vi "Picture Rotation.vi"(6 "Mask Color (Black)":u32(colorbox), 8 "transparent?":bool, 9 "theta (deg)":dbl(slide) scale=-180.0..180.0, 10 "image data in":T2, 11 "Path":path) -> (2 "image data out":T2, 3 "Picture":picture)   [LabVIEW 2018]
uses:
  <vilib>/picture/picture.llb/imagedata.ctl
  <vilib>/Utility/miscctls.llb/LVBoundsTypeDef.ctl
panel:
  out "output cluster":T1
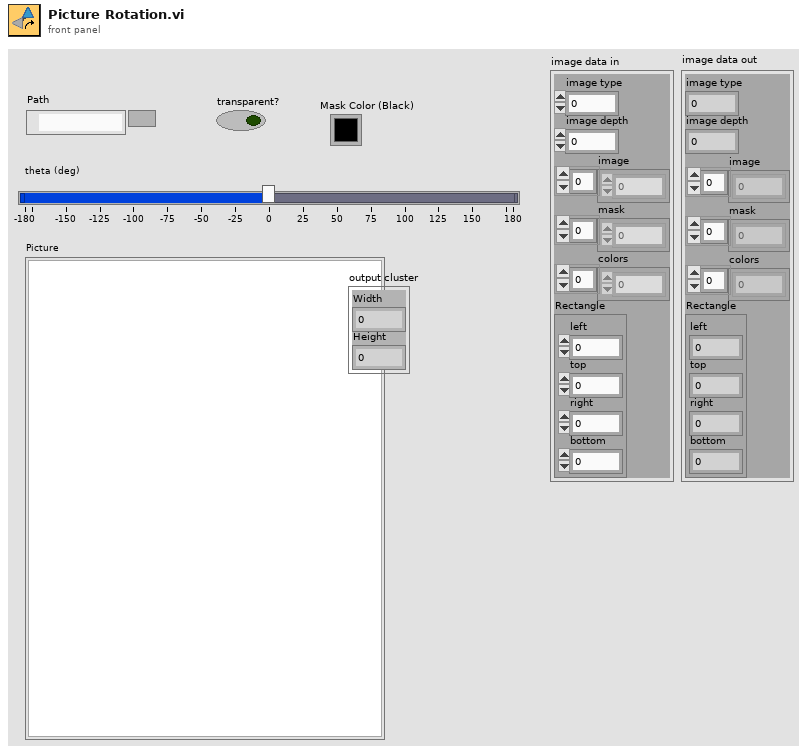
[diagram p1: front panel]
types:
  T1 = typedef "LVBoundsTypeDef.ctl" = cluster{"Width":u32, "Height":u32}
  T2 = typedef "imagedata.ctl" = cluster{"image type":i32, "image depth":i32, "image":u8[], "mask":u8[], "colors":u32[], "Rectangle":cluster{"left":i16, "top":i16, "right":i16, "bottom":i16}}
  T3 = cluster{"left":i16, "top":i16, "right":i16, "bottom":i16}
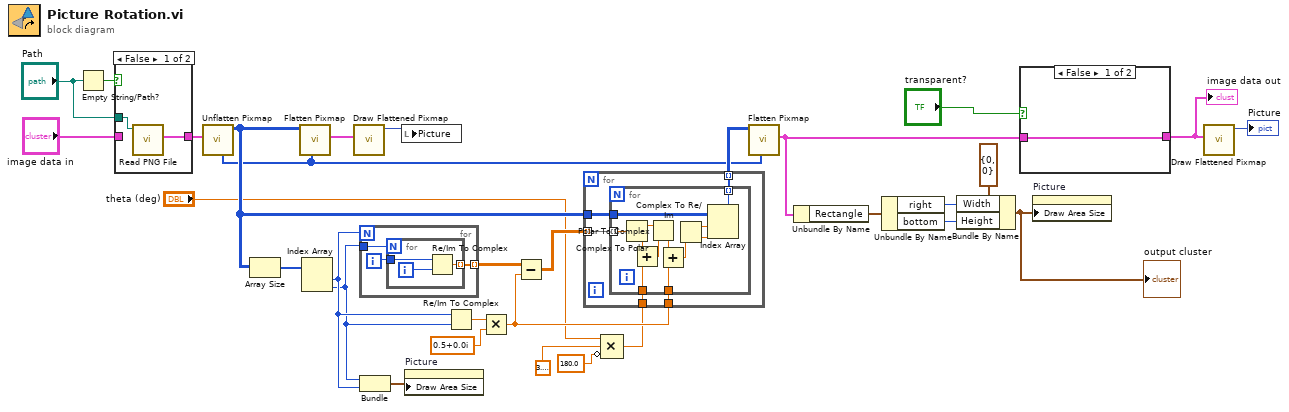
[diagram p0: block diagram]
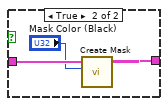
[diagram p2: hidden frame]
diagram:
  n1 = Empty String/Path?(string/path="Path") -> (empty?=w12:bool)
  n2 = case shown="False" w12 {
    tunnel: [w33 w34] -> w21
    tunnel: "Path" -> [w32 _]
    tunnel: "image data in" -> [_ w34]
    frame False {
      n3 = call <vilib>:"Read PNG File.vi"("path to PNG file"=w32) -> ("image data"=w33:T2)  [unwired: 8 in, 2 out]
    }
    frame True {
    }
  }
  n4 = call <vilib>:"Unflatten Pixmap.vi"("image data"=w21) -> ("24-bit pixmap"=w22:u32[][], "colors"=w19:u32[])  [unwired: 4 in, 5 out]
  n5 = Array Size(array=w22) -> (size(s)=w28:i32[])
  n6 = call <vilib>:"Flatten Pixmap.vi"("colors"=w19, "24-bit pixmap"=w22) -> ("image data"=w18:T2)  [unwired: 9 in]
  n7 = Index Array(array=w28) -> (element #1=w26:i32, element #2=w25:i32)  [unwired: 2 in]
  n8 = call <vilib>:"Draw Flattened Pixmap.vi"("image data"=w18) -> ("new picture"=w4:picture)  [unwired: 8 in]
  n9 = for {
    N: w26 -> [_]
    tunnel: w25 -> [w37]
    tunnel: [w35] -> w31 mode=indexing
    i -> [w36]
    n10 = for {
      N: w37 -> [_]
      tunnel: w36 -> [w39]
      tunnel: [w38] -> w35 mode=indexing
      i -> [w40]
      n11 = Re/Im To Complex(1:w40, 2:w39) -> (0:w38:cdb)
    }
  }
  n12 = Bundle(w25, w26) -> (w27:cluster{i32, i32})  [unwired: 1 in]
  n13 = local write "Picture"(w4) -> ()
  n14 = property on="Picture" class="Pict"("Draw Area Size"=w27) -> ()  [unwired: 2 in, 2 out]
  n15 = Re/Im To Complex(1:w25, 2:w26) -> (0:w29:cdb)
  n16 = Multiply(x=w29, y=cdb 0.5+0.0i) -> (x*y=w24:cdb)
  n17 = Subtract(x=w31, y=w24) -> (x-y=w30:cdb[][])
  n18 = Compound Arithmetic op=MULTIPLY("theta (deg)", 3.141592653589793, invert 180.0 ("value")) -> (w16:dbl)
  n19 = for {
    tunnel: w16 -> [w45]
    tunnel: w22 -> [w44]
    tunnel: w24 -> [w43]
    tunnel: w30 -> [w42] mode=indexing
    tunnel: [w41] -> w20 mode=indexing
    n20 = for {
      tunnel: w44 -> [w51]
      tunnel: w45 -> [w54]
      tunnel: w43 -> [w48]
      tunnel: w42 -> [w47] mode=indexing
      tunnel: [w46] -> w41 mode=indexing
      n21 = Complex To Polar(r * e^(i*theta)=w47) -> (r=w57:dbl, theta=w56:dbl)
      n22 = Add(x=w56, y=w54) -> (x+y=w55:dbl)
      n23 = Polar To Complex(1:w55, 2:w57) -> (0:w53:cdb)
      n24 = Add(x=w53, y=w48) -> (x+y=w49:cdb)
      n25 = Complex To Re/Im(x + iy=w49) -> (x=w52:dbl, y=w50:dbl)
      n26 = Index Array(array=w51, index (row)=w52, index (col)=w50) -> (element=w46:u32)
    }
  }
  n27 = call <vilib>:"Flatten Pixmap.vi"("colors"=w19, "24-bit pixmap"=w20) -> ("image data"=w8:T2)  [unwired: 9 in]
  n28 = Unbundle By Name(w8) -> ("Rectangle"=w7:T3)
  n29 = Unbundle By Name(w7) -> ("right"=w6:i16, "bottom"=w5:i16)
  n30 = Bundle By Name(cluster=T1 {"Width"=0, "Height"=0} ("Draw Area Size"), "Width"=w6, "Height"=w5) -> (w9:T1)
  "output cluster" <- w9
  n31 = case shown="False" "transparent?" {
    tunnel: w8 -> [w58 w61]
    tunnel: [w58 w60] -> w2
    frame False {
    }
    frame True {
      n32 = call <vilib>:"Create Mask.vi"("Mask Color (Black)"="Mask Color (Black)", "image data"=w61) -> ("image data"=w60:T2)  [unwired: 9 in]
    }
  }
  "image data out" <- w2
  n33 = property on="Picture" class="Pict"("Draw Area Size"=w9) -> ()  [unwired: 2 in, 2 out]
  n34 = call <vilib>:"Draw Flattened Pixmap.vi"("image data"=w2) -> ("new picture"=→"Picture":picture)  [unwired: 8 in]
